vi "Save 1PLOT.vi"(8 "error in (no error)":errorcluster, 10 "Refs":T1, 11 "Config Ops":T2={"file extension"="", "start path"=path ""}) -> (0 "error out":errorcluster)   [LabVIEW 2021, in "RocketPlot.lvlib"]
uses:
  RocketPlot.lvlib
  TypeDefs/Save 1PLOT config.ctl
  TypeDefs/Plot UI references.ctl
  Classes/RocketPlotHandle/RocketPlotHandle.lvclass
  <userlib>/bjustice/TipStripOOPanel/Classes/TipPanelHandle/TipPanelHandle.lvclass
  TypeDefs/Plot top row.ctl
  b42ebf4c-6e47-4da4-b815-0e84610f24a6.vi
  <vilib>/JDP Science/JSONtext/Variant to JSON Text.vi
  <vilib>/JDP Science/JSONtext/LVClass Serializer/JSONtext LVClass Serializer.lvclass
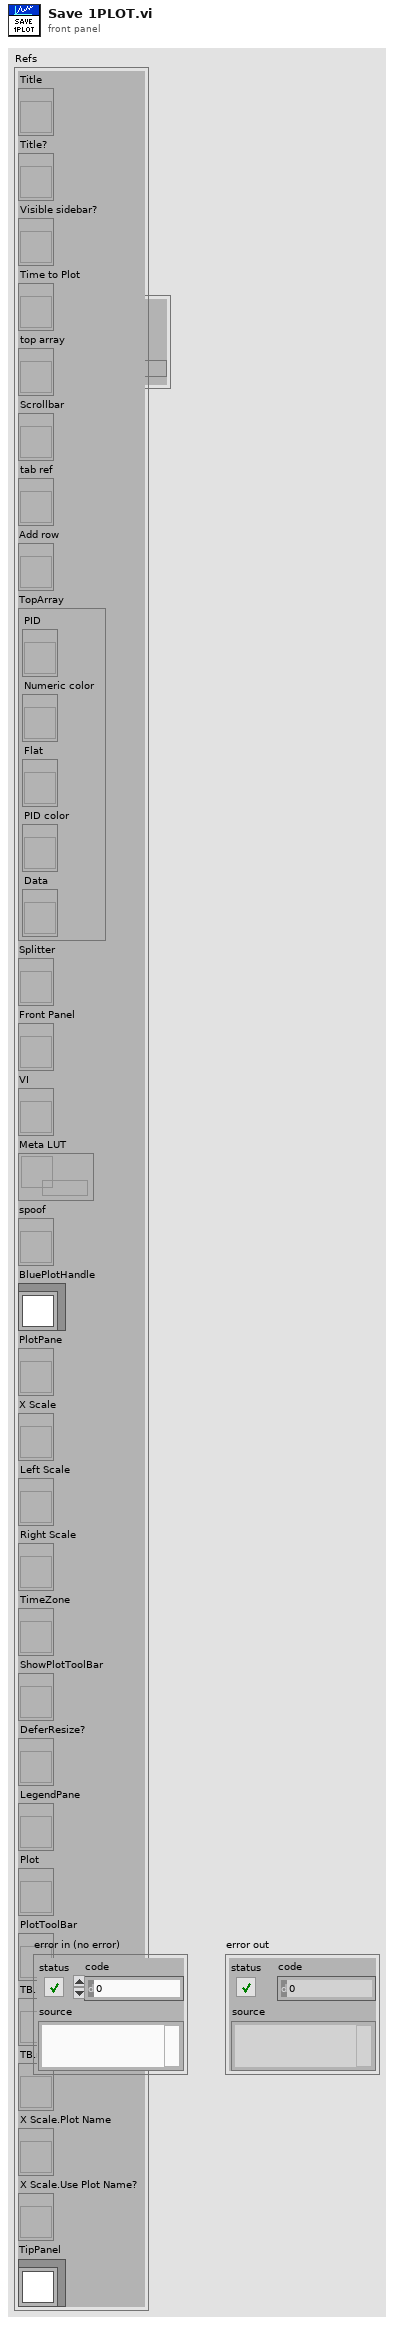
[diagram p1: front panel]
types:
  T1 = typedef "RocketPlot.lvlib/Plot UI references.ctl" = cluster{"Title":refnum<vi>, "Title?":refnum<vi>, "Visible sidebar?":refnum<vi>, "Time to Plot":refnum<vi>, "top array":refnum<vi>, "Scrollbar":refnum<vi>, "tab ref":refnum<vi>, "Add row":refnum<vi>, "TopArray":cluster{"PID":refnum<vi>, "Numeric color":refnum<vi>, "Flat":refnum<vi>, "PID color":refnum<vi>, "Data":refnum<vi>}, "Splitter":refnum<vi>, "Front Panel":refnum<vi>, "VI":refnum<vi>, "Meta LUT":refnum<data-value>, "spoof":refnum<vi>, "BluePlotHandle":refnum<class "RocketPlotHandle.lvclass">, "PlotPane":refnum<vi>, "X Scale":refnum<vi>, "Left Scale":refnum<vi>, "Right Scale":refnum<vi>, "TimeZone":refnum<vi>, "ShowPlotToolBar":refnum<vi>, "DeferResize?":refnum<vi>, "LegendPane":refnum<vi>, "Plot":refnum<vi>, "PlotToolBar":refnum<vi>, "TB.Info":refnum<vi>, "TB.max":refnum<vi>, "X Scale.Plot Name":refnum<vi>, "X Scale.Use Plot Name?":refnum<vi>, "TipPanel":refnum<class "TipPanelHandle.lvclass">}
  T2 = typedef "RocketPlot.lvlib/Save 1PLOT config.ctl" = cluster{"file extension":string, "start path":path}
  T3 = enum16{"open", "replace", "create", "open or create", "replace or create", "replace or create with confirmation"}
  T4 = typedef "RocketPlot.lvlib/plot load data V2.ctl" = cluster{"plots":T5[], "X-axis":T7, "Y-axes":T7[], "General":T8}
  T5 = typedef "RocketPlot.lvlib/plot properties V2.ctl" = cluster{"attributes":T6, "Numeric":dbl, "Flatline?":bool}
  T6 = typedef "RocketPlot.lvlib/plot attributes V2.ctl" = cluster{"Plot Color":u32, "Point Style":u8, "Line Style":u8, "Plot Interpolation":u8, "Line Width":u8, "Bar Plot Style":u8, "Fill To":i16, "X Scale Index":u32, "Y Scale Index":u32, "Anti-aliased":bool, "Label Format":u8, "Digital Transition Type":u8, "Digital Transition Location":u8, "Digital Line Style":u8, "Fill/Point Color":u32, "Plot Name":string, "Visible":bool}
  T7 = typedef "RocketPlot.lvlib/Plot scale axis properties.ctl" = cluster{"Name Label.Text":string, "Style":u8, "Tick Colors:Minor Tick Color":u32, "Tick Colors:Tick Color":u32, "Marker Colors:Text Color":u32, "Grid Colors:Major Color":u32, "Grid Colors:Minor Color":u32, "Mapping Mode":u8, "Flipped":bool, "Name Label.Visible":bool, "Name Label.Text Colors:Text Color":u32, "Scale Fit":u8, "Range:Maximum":dbl, "Range:Minimum":dbl, "Offset and Multiplier:Multiplier":dbl, "Offset and Multiplier:Offset":dbl, "Name Label.Font:Size":u32, "Marker.Font:Size":u32, "Uniform Marker Spacing?":bool, "Format String":string}
  T8 = typedef "RocketPlot.lvlib/Plot general properties.ctl" = cluster{"Title":string, "Time to Plot":dbl, "Title.Visible":bool, "Sidebar.Visible":bool, "Plot Area:Colors:BG Color":u32, "X Scale.Plot Name":string, "X Scale.Use Plot Name":bool}
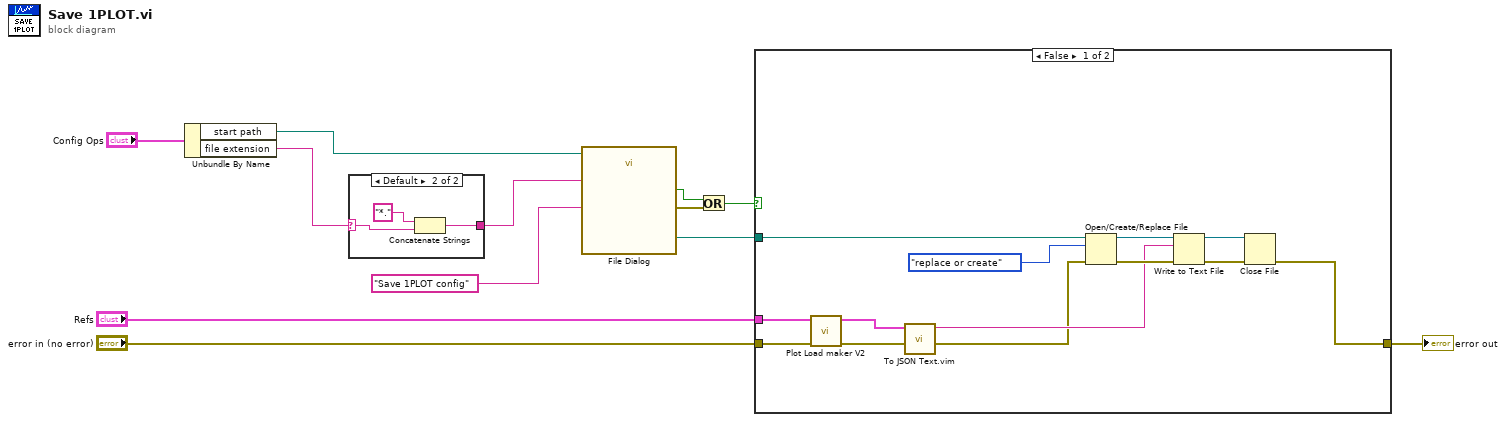
[diagram p0: block diagram]
diagram:
  n1 = Unbundle By Name("Config Ops") -> ("start path"=w11:path, "file extension"=w10:string)
  n2 = case shown="Default" w10 {
    selector: w10 -> [w13 w15]
    tunnel: [w13 w14] -> w9
    frame "" {
    }
    frame Default {
      n3 = Concatenate Strings("*." ("string"), w15) -> (w14:string)
    }
  }
  n4 = call "File Dialog"("start path"=w11, "prompt"="Save 1PLOT config", "pattern (all files)"=w9) -> ("selected path"=w4:path, "cancelled"=w7:bool, "error out"=w6:errorcluster)  [unwired: 9 in, 1 out]
  n5 = Or(x=w7, y=w6) -> (x .or. y?=w5:bool)
  n6 = case shown="False" w5 {
    tunnel: w4 -> [w21 _]
    tunnel: "Refs" -> [w29 _]
    tunnel: "error in (no error)" -> [w28 w30]
    tunnel: [w19 w30] -> w1
    frame False {
      n7 = call "Plot Load maker V2.vi"("error in (no error)"=w28, "Refs"=w29) -> ("error out"=w18:errorcluster, "Plot config"=w27:T4)  [unwired: 8 in]
      n8 = call "To JSON Text.vim"("error in (no error)"=w18, "Anything"=w27) -> ("error out"=w17:errorcluster, "<JSON>"=w20:string)  [unwired: 8 in]
      n9 = Open/Create/Replace File(file path (use dialog)=w21, error in=w17, operation (0:open)=T3."replace or create") -> (refnum out=w25:refnum<file>, error out=w23:errorcluster)  [unwired: 3 in, 1 out]
      n10 = Write to Text File(file (use dialog)=w25, text=w20, error in=w23) -> (refnum out=w24:refnum<file>, error out=w22:errorcluster)  [unwired: 1 in, 1 out]
      n11 = Close File(refnum=w24, error in=w22) -> (error out=w19:errorcluster)  [unwired: 1 out]
    }
    frame True {
    }
  }
  "error out" <- w1
